vi "subGetItemInfos.vi"(11 "Path":path) -> (1 "Project refs":refnum<vi>[](array[refnum]), 2 "Local Host App Instance":refnum<vi>, 3 "Item info":T1)   [LabVIEW 2020, in "SolutionBuilder.lvlib"]
uses:
  SolutionBuilder.lvlib
  ItemInfo.ctl
  ProjectInfo.ctl
  FileInfo.ctl
  b6d37d69-d619-4dba-9ed7-0923f92a2504.vi
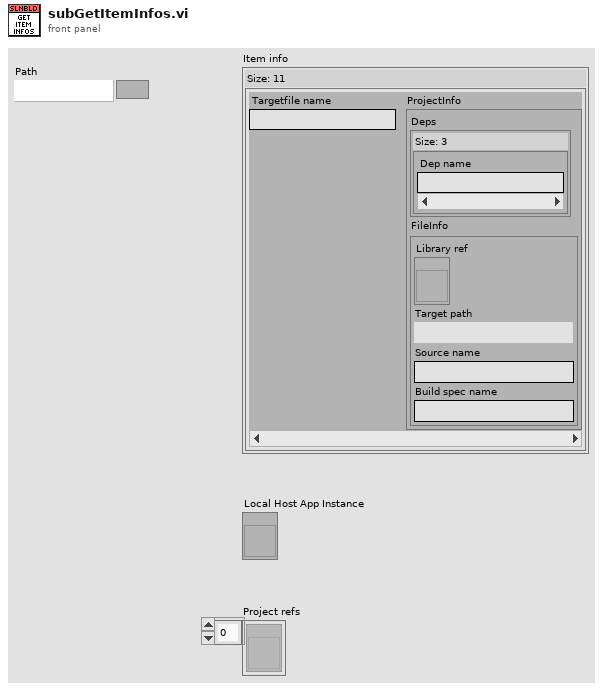
[diagram p1: front panel]
types:
  T1 = typedef "SolutionBuilder.lvlib/ItemInfo.ctl" = map{string, T2}
  T2 = typedef "SolutionBuilder.lvlib/ProjectInfo.ctl" = cluster{"Deps":set{string}, "FileInfo":T3}
  T3 = typedef "SolutionBuilder.lvlib/FileInfo.ctl" = cluster{"Library ref":refnum<vi>, "Target path":path, "Source name":string, "Build spec name":string}
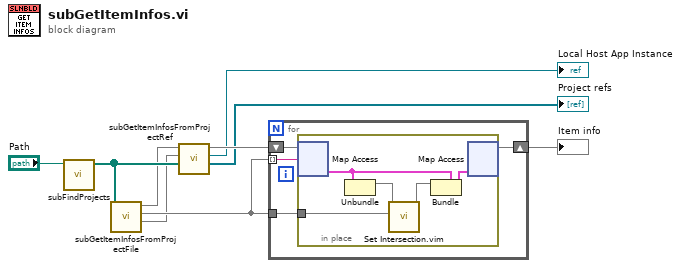
[diagram p0: block diagram]
diagram:
  n1 = call "subFindProjects.vi"("Path"="Path") -> ("All Files in Dir"=w6:path[])  [unwired: 10 in]
  n2 = call "subGetItemInfosFromProjectFile.vi"("All Files in Dir"=w6) -> ("Source dist"=w1:map{string, set{string}}, "TargetFile name"=w8:set{string}, "TargetFile info"=w5:T1)  [unwired: 8 in]
  n3 = call "subGetItemInfosFromProjectRef.vi"("All Files in Dir"=w6, "Source dist"=w1, "TargetFile info in"=w5) -> ("Project refs"=→"Project refs":refnum<vi>[], "Local Host App Instance"=→"Local Host App Instance":refnum<vi>, "TargetFile info"=w4:T1)  [unwired: 6 in]
  n4 = for {
    tunnel: w8 -> [w13]
    tunnel: w8 -> [w11] mode=indexing
    shift-right: [w10] -> w9
    shift-left: w4 -> [w12]
    n5 = in-place {
      in-place-border: w13 -> [w17]
      n6 = in-place-map #1(w12, w11) -> (w14:T2)  [unwired: 1 in, 1 out]
      n7 = Unbundle(w14) -> ("Deps"=w18:set{string})  [unwired: 1 out]
      n8 = call "Set Intersection.vim"("set 2"=w17, "set 1"=w18) -> ("intersection"=w16:set{string})  [unwired: 9 in]
      n9 = Bundle(cluster=w14, "Deps"=w16) -> (w15:T2)  [unwired: 1 in]
      n10 = in-place-map #1(w15) -> (w10:T1)  [unwired: 1 in, 2 out]
    }
  }
  "Item info" <- w9
